vi "CCD Get Config.vi"(8 "error in (no error)":errorcluster, 11 "CCD in":refnum<class "CCD.lvclass">) -> (0 "error out":errorcluster, 2 "config data":T1={"centerWavelength"=0.0, "chipHSpacing"=0.0, "chipHeight"=0.0, "chipName"="$.configuration", "chipSerialNumber"="$.configuration", "chipVSpacing"=0.0, "chipWidth"=0.0, "deviceType"="$.configuration", "fitParameters"=[], "gains"=[], "hardwareAvgAvailable"=FALSE, "lineScan"=FALSE, "productId"="$.configuration", "serialNumber"="", "signals"=[], "speeds"=[], "supportedFeatures"={"cf_3PositionSlit"=FALSE, "cf_CMOSOffsetCorrection"=FALSE, "cf_Cleaning"=FALSE, "cf_DSP"=FALSE, "cf_DSPBin2X"=FALSE, "cf_DelayAfterTrigger"=FALSE, "cf_Delays"=FALSE, "cf_EMCCD"=FALSE, "cf_EShutter"=FALSE, "cf_HDR"=FALSE, "cf_Image"=FALSE, "cf_MemorySlots"=FALSE, "cf_Metadata"=FALSE, "cf_MultipleExposeTimes"=FALSE, "cf_MultipleSensors"=FALSE, "cf_PulseSummation"=FALSE, "cf_ROIs"=FALSE, "cf_Signals"=FALSE, "cf_Spectra"=FALSE, "cf_TriggerQualifier"=FALSE, "cf_Triggers"=FALSE}, "triggers"=[], "version"=""}, 3 "CCD out":refnum<class "CCD.lvclass">)   [LabVIEW 2020, in "Examples.lvlib"]
uses:
  Examples.lvlib
  Classes/CCD/CCD.lvclass
  Classes/CCD/Gain.ctl
  Classes/CCD/Speed.ctl
  Classes/CCD/Type.ctl
  Classes/CCD/Event.ctl
  Classes/CCD/Signal.ctl
  Classes/CCD/Trigger.ctl
  Classes/CCD/SupportedFeatures.ctl
  Classes/CCD/GetConfig.ctl
panel:
  # "Connector Pane"
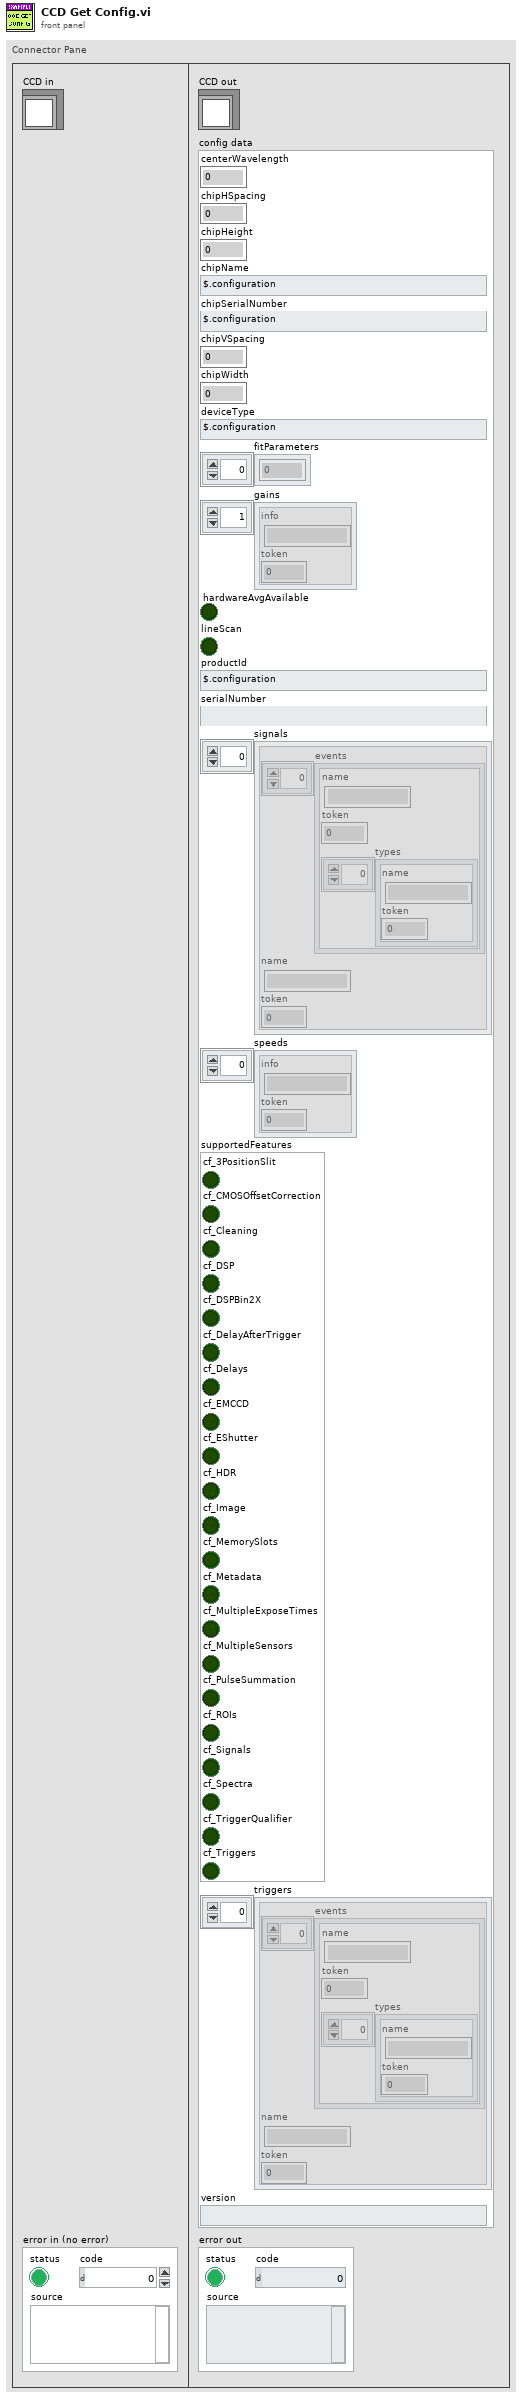
[diagram p1: front panel]
types:
  T1 = typedef "horiba.lvlib/CCD.lvclass/GetConfig.ctl" = cluster{"centerWavelength":dbl, "chipHSpacing":dbl, "chipHeight":dbl, "chipName":string, "chipSerialNumber":string, "chipVSpacing":dbl, "chipWidth":dbl, "deviceType":string, "fitParameters":dbl[], "gains":T2[], "hardwareAvgAvailable":bool, "lineScan":bool, "productId":string, "serialNumber":string, "signals":T3[], "speeds":T6[], "supportedFeatures":T7, "triggers":T8[], "version":string}
  T2 = typedef "horiba.lvlib/CCD.lvclass/Gain.ctl" = cluster{"info":string, "token":i32}
  T3 = typedef "horiba.lvlib/CCD.lvclass/Signal.ctl" = cluster{"events":T4[], "name":string, "token":i32}
  T4 = typedef "horiba.lvlib/CCD.lvclass/Event.ctl" = cluster{"name":string, "token":i32, "types":T5[]}
  T5 = typedef "horiba.lvlib/CCD.lvclass/Type.ctl" = cluster{"name":string, "token":i32}
  T6 = typedef "horiba.lvlib/CCD.lvclass/Speed.ctl" = cluster{"info":string, "token":i32}
  T7 = typedef "horiba.lvlib/CCD.lvclass/SupportedFeatures.ctl" = cluster{"cf_3PositionSlit":bool, "cf_CMOSOffsetCorrection":bool, "cf_Cleaning":bool, "cf_DSP":bool, "cf_DSPBin2X":bool, "cf_DelayAfterTrigger":bool, "cf_Delays":bool, "cf_EMCCD":bool, "cf_EShutter":bool, "cf_HDR":bool, "cf_Image":bool, "cf_MemorySlots":bool, "cf_Metadata":bool, "cf_MultipleExposeTimes":bool, "cf_MultipleSensors":bool, "cf_PulseSummation":bool, "cf_ROIs":bool, "cf_Signals":bool, "cf_Spectra":bool, "cf_TriggerQualifier":bool, "cf_Triggers":bool}
  T8 = typedef "horiba.lvlib/CCD.lvclass/Trigger.ctl" = cluster{"events":T4[], "name":string, "token":i32}
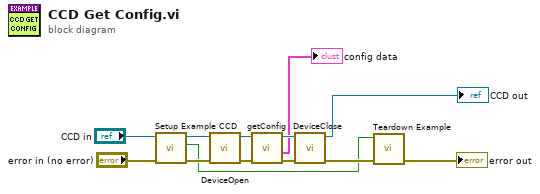
[diagram p0: block diagram]
diagram:
  n1 = call "Setup Example CCD.vi"("error in (no error)"="error in (no error)", "CCD in"="CCD in") -> ("error out"=w8:errorcluster, "Module Was Already Running?"=w2:bool, "CCD out"=w4:refnum<class "CCD.lvclass">)  [unwired: 7 in]
  n2 = call-dynamic "DeviceOpen.vi"("error in (no error)"=w8, "CCD in"=w4) -> ("error out"=w13:errorcluster, "CCD out"=w9:refnum<class "CCD.lvclass">)  [unwired: 6 in, 2 out]
  n3 = call "getConfig.vi"("error in (no error)"=w13, "CCD in"=w9) -> ("error out"=w12:errorcluster, "config data"=→"config data":T1, "CCD out"=w10:refnum<class "CCD.lvclass">)  [unwired: 6 in, 1 out]
  n4 = call-dynamic "DeviceClose.vi"("error in (no error)"=w12, "CCD in"=w10) -> ("error out"=w5:errorcluster, "CCD out"=→"CCD out":refnum<class "CCD.lvclass">)  [unwired: 5 in, 3 out]
  n5 = call "Teardown Example.vi"("error in (no error)"=w5, "Module Was Already Running?"=w2) -> ("error out"=→"error out":errorcluster)  [unwired: 9 in]
